vi "Check Struct from Variant.vi"(10 "Type Constructor":T1, 11 "variant":variant) -> (0 "error out":errorcluster, 1 "BaseType":T3, 2 "Is Struct?":bool, 3 "Shape":T2, 4 "Is Char Array?":bool, 5 "Is Struct with valid fieldnames?":bool, 7 "Invalid Fieldnames":string[](array[string]))   [LabVIEW 2021, in "MathScriptCompiler.lvlib"]
uses:
  <vilib>/imath/engines/lvmath2/MathScriptCompiler/MathScriptCompiler.llb/MathScriptCompiler.lvlib
  <vilib>/imath/engines/lvmath/Functions/Error Handling/error.ctl
  <vilib>/imath/engines/lvmath2/MathScriptCompiler/Type/BaseEltType.llb/BaseType.ctl
  <vilib>/imath/engines/lvmath2/MathScriptCompiler/Type/Matrix.llb/Shape.ctl
  <vilib>/imath/engines/lvmath2/MathScriptCompiler/MathScriptTypes.llb/ConstructorsType.ctl
  <vilib>/imath/engines/lvmath2/MathScriptCompiler/Type/StrictType.llb/StrictType.lvclass
  <vilib>/imath/engines/lvmath2/MathScriptCompiler/MathScriptTypes.llb/MathScriptTypes.lvlib
  <vilib>/imath/engines/lvmath2/MathScriptCompiler/Type/StructEltType.llb/StructEltType.lvclass
  <vilib>/imath/engines/lvmath2/MathScriptCompiler/Type/BaseEltType.llb/BaseEltType.lvclass
  <vilib>/imath/engines/lvmath2/MathScriptCompiler/Type/Matrix.llb/Matrix.lvclass
panel:
  out "Type String":string
  out "Error Enum":T4
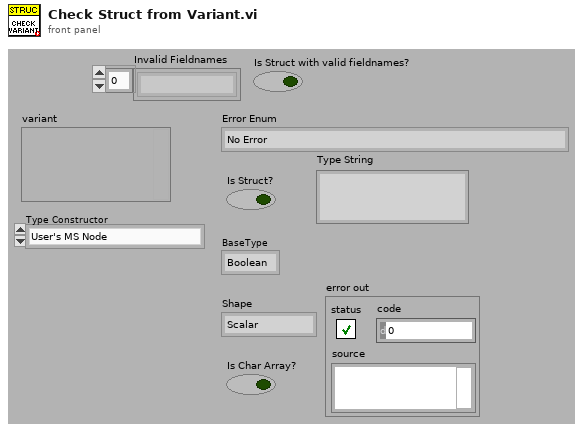
[diagram p1: front panel]
types:
  T1 = typedef "MathScriptTypes.lvlib/ConstructorsType.ctl" = enum16{"User's MS Node", "UDF MS Node", "BIF Output", "Window Mode Output", "Window Mode Input", "BIF Input"}
  T2 = typedef "MathScriptTypes.lvlib/Matrix.lvclass/Shape.ctl" = enum16{"Scalar", "Row Vector", "Column Vector", "Matrix"}
  T3 = typedef "MathScriptTypes.lvlib/BaseEltType.lvclass/BaseType.ctl" = enum16{"Boolean", "U8", "U16", "U32", "U64", "I8", "I16", "I32", "I64", "SGL", "DBL", "EXT", "CSG", "CDB", "CXT"}
  T4 = typedef "error.ctl" = enum16{"No Error", "Problem", "Input type must not be void", "Incorrect number of parameters", "Function not defined for non-numeric types", "An output variable of the user-defined function is undefined", "Function only defined for character arrays", "Function not defined for boolean, character, or single precision", "Function not defined for complex types", "Not a valid operation", "Inputs must be scalar", "Input matrices are not the same size", "Function only available on RT", "Input matrices must be nonnegative integers of the same type", "Arguments must be non-negative integers less than bitmax", "Number to complement must be less than 2^N", "Bit to get is outside range", "Bit to set is outside range", "Input must be real type ", "At least one parameter must be scalar", "Unable to display plug-in data on RT", "Function not defined for higher dimensional matrices", "Invalid attributes", "Wrong Type of Input Arguments", "Wrong Argument Option", "Invalid file identifier", "Indices must be real positive integers", "The variable is not a matrix data type.", "Number of elements must be the same for indices and values", "You cannot replace elements of a matrix with non-matrix data types.", "Cannot resize a 2D matrix with a linear index", "Unknown variable or symbol", "Indices out of range", "Empty matrix deletion can not be used with two indices", "Number of rows and columns must be the same for indices and values.", "Complex cannot be converted to Boolean", "Char cannot be converted to Boolean", "int64 cannot be converted to Boolean", "uint64 cannot be converted to Boolean", "You cannot convert a Boolean to a character.", "Incompatible input size in 3D surface function", "All rows must have the same number of columns", "Incompatible types", "Invalid matrix dimensions", "Dimension must be 1 or 2", "Base must be an integer between 2 and 36", "Invalid input", "Square matrix required", "Function 'timerstart' must be called before 'timerstop'", "Arguments must be positive real", "Step must not be zero", "Wrong number of input arguments", "Wrong number of output arguments", "Too many index arguments", "Input scalar must be >= 0", "Input scalar must be positive", "Input scalar must not be 0", "Input scalar must be in range [0,1]", "Can't use conditionally defined variable that's undefined", "Input must be a vector", "RT Exec Trace Toolkit not licensed", "Empty vector error", "All elements must be in domain [-1,1]", "All real elements of input vector must be >= 0", "All elements of input vector must be positive", "Values of input vectors are not compatible", "DAQmx not installed", "Input vector must be an increasing vector", "Dereferenced field does not exist within the struct", "A vector or matrix of structures must be indexed before it can be dereferenced", "Lenths of two input vectors are not compatible", "Invalid fieldname", "Empty matrix error", "Cannot use '.' on a type other than Struct", "Unused074", "Data type of the struct's field name is invalid", "Using . to dereference data that is not a struct", "Input struct contains invalid type ", "Size of input matrix is incompatible with input size", "Invalid format specifier", "Could not find field within struct", "Bad permutation array", "Mismatched fieldnames", "ode: User Function could not be opened", "ode: User Function signature does not meet ode requirements", "Unused085", "RunTime: MathScript could not be compiled", "Unknown function", "Only scalars and strings supported", "ode: User Function signature has incorrect number of inputs", "ode:User Function signature has incorrect number of outputs", "Range is too large", "End used without variable", "Function not available (RTE)", "Custom user error", "Arguments must be integers less than bitmax", "Shared library not found", "Header file not found", "Shared library already loaded", "Shared library not loaded", "Shared library function not found", "Shared library string return problem", "Problem calling shared library function", "Problem loading shared library from OS", "Problem parsing shared library header file", "Shared library incompatible types", "Shared library unsupported return type", "Shared library function not exported", "Shared library unsupported input type", "Problem unloading shared library from OS", "Function only available from UI", "Function specified in argument is missing", "An internal error has occurred", "Invalid object", "Invalid property", "Read-only property", "A break command has occurred", "A continue command has occurred", "A return command has occurred", "ode: times parameter invalid", "Function specified in argument has incorrect signature", "Function not found in file", "Reserved keyword cannot be defined as variable", "Reserved keyword cannot be defined as a function or script", "Arguments must be string literals", "Function not supported on this platform", "All columns must have the same number of rows", "Function ignored in RTE warning", "Cannot use : as a parameter that is not a variable", "Output can't be coerced to requested type", "Function not supported on current target", "Variable dependent on an unwired function input", "Unused132", "Unused133", "Unused134", "Unused135", "Unused136", "Unused137", "Unused138", "Unused139", "Global/Persistent must only take constants as arguments.", "Varargin must be last input in the function definition.", "Varargout must be last output in the function definition.", "Invalid output type. Cannot output a cell array of any type other than string.", "Invalid output type. Type is a dynamic struct.", "Invalid output type. Type is a struct that has a field whose type is not known until run-time", "Invalid output type. Type is a struct that has a field which is a plot object.", "MathScript parser DLL missing", "MathScript requires LabVIEW Full", "MathScript license is invalid or missing", "Varargout not supported except in assignments."}
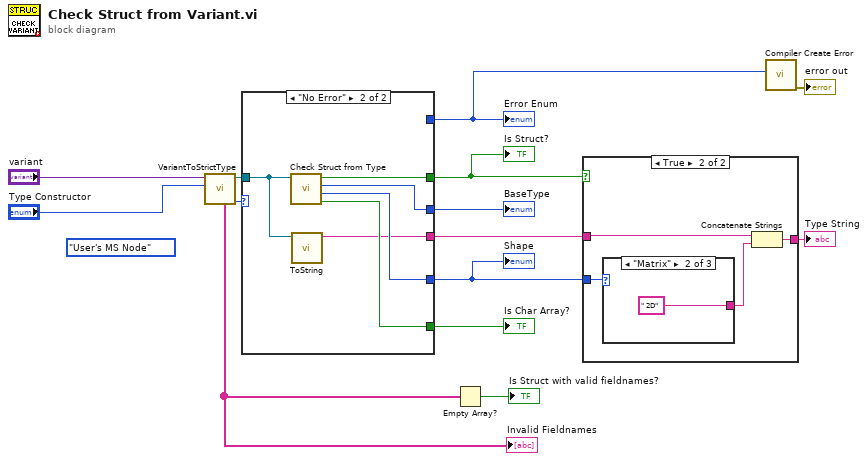
[diagram p0: block diagram]
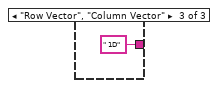
[diagram p4: hidden frame]
diagram:
  (unwired) ConstructorsType."User's MS Node" ("Enum")
  n1 = call <vilib>:"VariantToStrictType.vi"("Enum"="Type Constructor", "Variant(*)"="variant") -> ("Error Enum"=w13:T4, "StrictType"=w10:refnum<class "StrictType.lvclass">, "Invalid Fieldnames out"=w2:string[])  [unwired: 6 in, 1 out]
  "Invalid Fieldnames" <- w2
  n2 = case shown="\"No Error\"" w13 {
    selector: w13 -> [w15 _]
    tunnel: w10 -> [_ w17]
    tunnel: [_ w21] -> w7
    tunnel: [_ w20] -> w11
    tunnel: [_ w19] -> w9
    tunnel: [_ w18] -> w12
    tunnel: [w15 _] -> w5
    tunnel: [_ w16] -> w8
    frame Default {
    }
    frame "No Error" {
      n3 = call <vilib>:"Check Struct from Type.vi"("StrictType"=w17) -> ("Is Char Array?"=w20:bool, "Shape"=w21:T2, "BaseType"=w18:T3, "Is Struct?"=w19:bool)  [unwired: 6 in, 1 out]
      n4 = call-dynamic "ToString.vi"("Type.lvclass"=w17) -> ("String"=w16:string)  [unwired: 10 out]
    }
  }
  "Error Enum" <- w5
  "BaseType" <- w12
  "Is Struct?" <- w9
  "Is Char Array?" <- w11
  "Shape" <- w7
  n5 = Empty Array?(array=w2) -> (empty?=→"Is Struct with valid fieldnames?":bool)
  n6 = case shown="True" w9 {
    tunnel: w8 -> [_ w24]
    tunnel: w7 -> [_ w25]
    tunnel: [_ w23] -> w6
    frame False {
    }
    frame True {
      n7 = case shown="\"Matrix\"" w25 {
        tunnel: [_ " 2D" ("string") " 1D" ("string")] -> w22
        frame "Scalar", Default {
        }
        frame "Matrix" {
        }
        frame "Row Vector", "Column Vector" {
        }
      }
      n8 = Concatenate Strings(w24, w22) -> (w23:string)
    }
  }
  "Type String" <- w6
  n9 = call <vilib>:"Compiler Create Error.vi"("Error Enum"=w5) -> ("error out"=→"error out":errorcluster)  [unwired: 10 in]
